vi "String2Bool.vi"(7 "String":string) -> (3 "Boolean":bool)   [LabVIEW 2024]
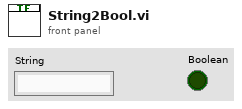
[diagram p1: front panel]
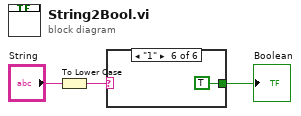
[diagram p0: block diagram]
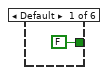
[diagram p2: hidden frame]
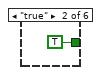
[diagram p3: hidden frame]
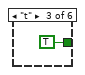
[diagram p4: hidden frame]
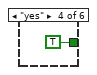
[diagram p5: hidden frame]
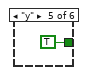
[diagram p6: hidden frame]
diagram:
  n1 = To Lower Case(string="String") -> (all lower case string=w1:string)
  n2 = case shown="\"1\"" w1 {
    tunnel: [FALSE TRUE TRUE TRUE TRUE TRUE] -> w2
    frame Default {
    }
    frame "true" {
    }
    frame "t" {
    }
    frame "yes" {
    }
    frame "y" {
    }
    frame "1" {
    }
  }
  "Boolean" <- w2
